vi "DeCoF extract mulit-component binary.vi"(2 "decoded binary blob":string, 3 "identifier":string) -> (0 "bytes":u8[](array[numeric]), 1 "found":bool)   [LabVIEW 2013]
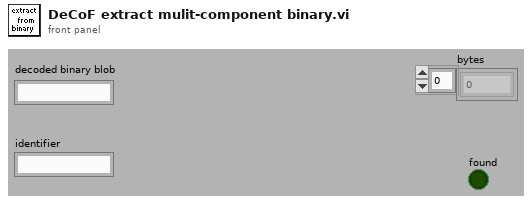
[diagram p1: front panel]
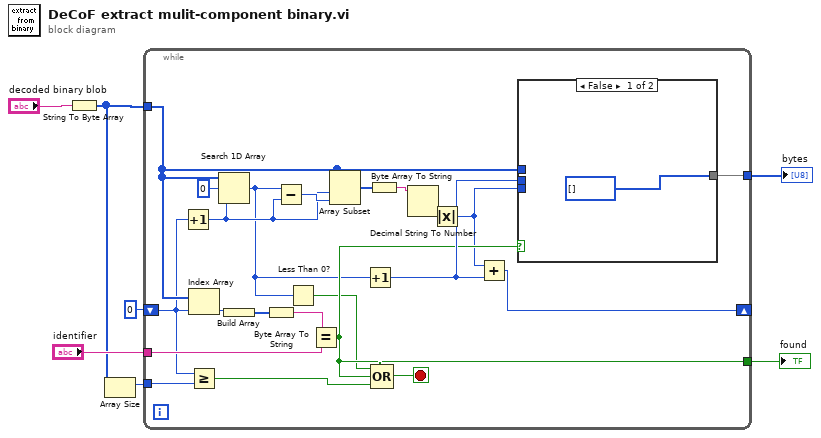
[diagram p0: block diagram]
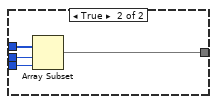
[diagram p2: hidden frame]
diagram:
  n1 = String To Byte Array(string="decoded binary blob") -> (unsigned byte array=w3:u8[])
  n2 = Array Size(array=w3) -> (size(s)=w2:i32)
  n3 = while {
    tunnel: w3 -> [w23]
    shift-right: [w11] -> _
    shift-left: 0 -> [w13]
    tunnel: "identifier" -> [w19]
    tunnel: [w14] -> w4
    tunnel: [w18] -> w1
    tunnel: w2 -> [w17]
    stop <- w15 stop-if-true
    n4 = Increment(x=w13) -> (x+1=w12:i32)
    n5 = Index Array(array=w23, index=w13) -> (element=w29:u8)
    n6 = Greater Or Equal?(x=w13, y=w17) -> (x >= y?=w16:bool)
    n7 = Search 1D Array(1D array=w23, element=u8 0, start index (0)=w12) -> (index of element=w9:i32)
    n8 = Build Array(w29) -> (w28:u8[])
    n9 = Byte Array To String(unsigned byte array=w28) -> (string=w20:string)
    n10 = Subtract(x=w9, y=w12) -> (x-y=w24:i32)
    n11 = Less Than 0?(x=w9) -> (x < 0?=w8:bool)
    n12 = Equal?(x=w20, y=w19) -> (x = y?=w14:bool)
    n13 = Array Subset(array=w23, index=w12, length=w24) -> (w26:u8[])
    n14 = Increment(x=w9) -> (x+1=w22:i32)
    n15 = Byte Array To String(unsigned byte array=w26) -> (string=w25:string)
    n16 = Compound Arithmetic op=OR(w8, w14, w16) -> (w15:bool)
    n17 = Decimal String To Number(string=w25) -> (number=w21:i32)  [unwired: 2 in, 1 out]
    n18 = Absolute Value(x=w21) -> (abs(x)=w10:i32)
    n19 = Add(x=w10, y=w22) -> (x+y=w11:i32)
    n20 = case shown="False" w14 {
      tunnel: w23 -> [_ w34]
      tunnel: w22 -> [_ w33]
      tunnel: w10 -> [_ w32]
      tunnel: [u8[] [] w31] -> w18
      frame False {
      }
      frame True {
        n21 = Array Subset(array=w34, index=w33, length=w32) -> (w31:u8[])
      }
    }
  }
  "found" <- w4
  "bytes" <- w1
